vi "FolderMon control.vi"(4 "error in (no error)":errorcluster, 6 "Polling (-1:  Unchanged)":i32=-1, 7 "Action (START)":enum16{"START", "STOP"}(ring)) -> (0 "error out":errorcluster)   [LabVIEW 2011]
uses:
  FolderMon config.ctl
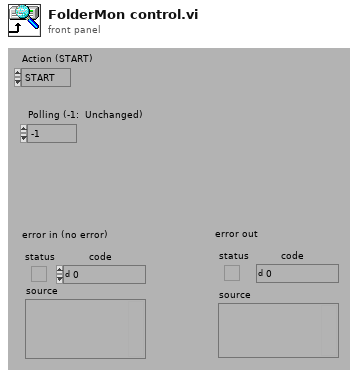
[diagram p1: front panel]
types:
  T1 = typedef "FolderMon config.ctl" = cluster{"Monitoring Folder":path, "Callback VI":string}
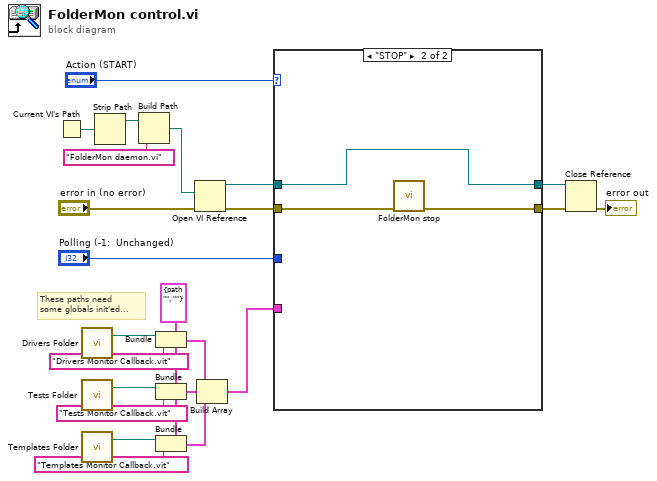
[diagram p0: block diagram]
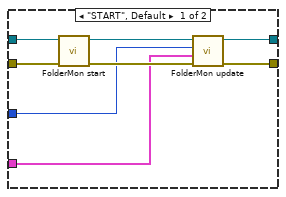
[diagram p2: hidden frame]
diagram:
  w2 = T1 {"Monitoring Folder"=path "", "Callback VI"=""} ("Monitor")
  # "These paths need\nsome globals init'ed..."
  n1 = Current VI's Path() -> (path=w22:path)
  n2 = call "Drivers Folder.vi"() -> ("Drivers Folder"=w11:path)  [unwired: 1 in, 2 out]
  n3 = call "Tests Folder.vi"() -> ("Tests Folder"=w10:path)  [unwired: 1 in, 2 out]
  n4 = call "Templates Folder.vi"() -> ("Templates Folder"=w9:path)  [unwired: 1 in, 2 out]
  n5 = Strip Path(path=w22) -> (stripped path=w21:path)  [unwired: 1 out]
  n6 = Build Path(base path=w21, name or relative path="FolderMon daemon.vi") -> (appended path=w19:path)
  n7 = Bundle(cluster=w2, "Monitoring Folder"=w11, "Callback VI"="Drivers Monitor Callback.vit" ("username (\"\")")) -> (w7:T1)
  n8 = Bundle(cluster=w2, "Monitoring Folder"=w10, "Callback VI"="Tests Monitor Callback.vit" ("username (\"\")")) -> (w8:T1)
  n9 = Bundle(cluster=w2, "Monitoring Folder"=w9, "Callback VI"="Templates Monitor Callback.vit" ("username (\"\")")) -> (w6:T1)
  n10 = Open VI Reference(vi path=w19, error in (no error)="error in (no error)") -> (vi reference=w18:refnum<vi>, error out=w17:errorcluster)  [unwired: 4 out]
  n11 = Build Array(w7, w8, w6) -> (w1:T1[])
  n12 = case shown="\"STOP\"" "Action (START)" {
    tunnel: w18 -> [w31 w32]
    tunnel: w17 -> [w30 w34]
    tunnel: "Polling (-1:  Unchanged)" -> [w28 _]
    tunnel: [w26 w32] -> w15
    tunnel: [w25 w33] -> w14
    tunnel: w1 -> [w24 _]
    frame "START", Default {
      n13 = call "FolderMon start.vi"("error in (no error)"=w30, "daemon VI ref"=w31) -> ("error out"=w29:errorcluster, "dup daemon VI ref"=w27:refnum<vi>)  [unwired: 4 out]
      n14 = call "FolderMon update.vi"("error in (no error)"=w29, "FolderMonitoring"=w24, "Polling (-1:  Unchanged)"=w28, "daemon VI Ref"=w27) -> ("error out"=w25:errorcluster, "dup daemon VI Ref"=w26:refnum<vi>)  [unwired: 2 out]
    }
    frame "STOP" {
      n15 = call "FolderMon stop.vi"("error in (no error)"=w34) -> ("error out"=w33:errorcluster)  [unwired: 6 out]
    }
  }
  n16 = Close Reference(reference=w15, error in (no error)=w14) -> (error out=→"error out":errorcluster)
